vi "Write.vi"(0 "reference in":refnum<class "ConfigInterface.lvclass">, 5 "Data":variant, 7 "Name":string, 11 "error in (no error)":errorcluster) -> (4 "reference out":refnum<class "ConfigInterface.lvclass">, 6 "Data dub":variant, 8 "Name dub":string, 15 "error out":errorcluster)   [LabVIEW 2019, in "ConfigInterface.lvclass"]
uses:
  ConfigInterface.lvclass
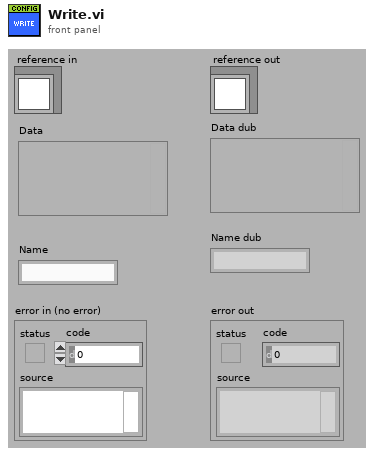
[diagram p1: front panel]
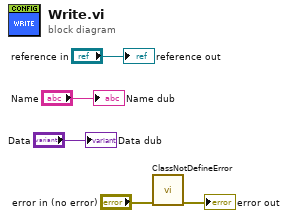
[diagram p0: block diagram]
diagram:
  n1 = call "ClassNotDefineError.vi"("error in (no error)"="error in (no error)") -> ("error out"=→"error out":errorcluster)  [unwired: 14 in]
  "reference out" <- "reference in"
  "Name dub" <- "Name"
  "Data dub" <- "Data"
